vi "XPS_single_axis_control.vi"() -> ()   [LabVIEW 2015]
panel:
  in  "STOP?":bool=TRUE
  out "Current Position":dbl format="%#_13g"
  out "Axis One Position":dbl(graph)
  in  "Target Position":dbl format="%#_13g"
  in  "Group Name":string
  in  "IP Address":string
  # "IP Address of the XPS controller\nis fixed to 192.168.1.43"
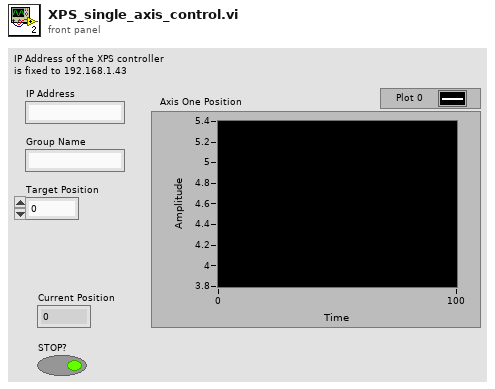
[diagram p1: front panel]
types:
  T1 = cluster{"connection TCP":refnum<k5>, "LogTo File":bool, "Log File refnum":refnum<file>, "no error if error log":bool}
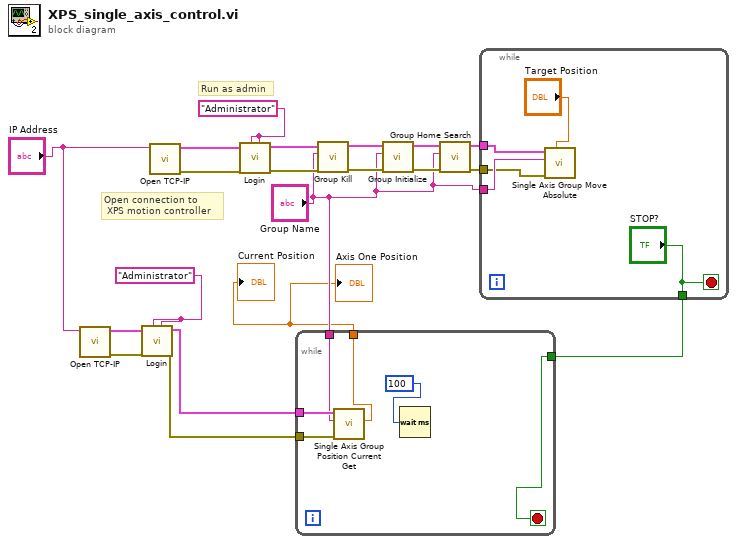
[diagram p0: block diagram]
diagram:
  w6 = "Administrator"
  w19 = "Administrator"
  # "Run as admin"
  # "Open connection to\n XPS motion controller"
  n1 = call <userlib>:"Open TCP-IP.vi"("IP address"="IP Address") -> ("error out"=w7:errorcluster, "Connection ID"=w8:T1)  [unwired: 8 in, 1 out]
  n2 = call <userlib>:"Login.vi"("Password"=w6, "User"=w6, "error in (no error)"=w7, "connection ID in"=w8) -> ("error out"=w4:errorcluster, "connection ID out"=w5:T1)  [unwired: 5 in, 1 out]
  n3 = call <userlib>:"Open TCP-IP.vi"("IP address"="IP Address") -> ("error out"=w14:errorcluster, "Connection ID"=w20:T1)  [unwired: 8 in, 1 out]
  n4 = call <userlib>:"Login.vi"("Password"=w19, "User"=w19, "error in (no error)"=w14, "connection ID in"=w20) -> ("error out"=w13:errorcluster, "connection ID out"=w18:T1)  [unwired: 5 in, 1 out]
  n5 = call <userlib>:"Group Kill.vi"("error in (no error)"=w13, "Group Name (250 c max)"="Group Name", "connection ID in"=w18) -> ("error out"=w12:errorcluster, "connection ID out"=w17:T1)  [unwired: 6 in, 1 out]
  n6 = call <userlib>:"Group Initialize.vi"("error in (no error)"=w12, "Group Name (250 c max)"="Group Name", "connection ID in"=w17) -> ("error out"=w11:errorcluster, "connection ID out"=w16:T1)  [unwired: 6 in, 1 out]
  n7 = call <userlib>:"Group Home Search.vi"("error in (no error)"=w11, "Group Name (250 c max)"="Group Name", "connection ID in"=w16) -> ("error out"=w10:errorcluster, "connection ID out"=w15:T1)  [unwired: 6 in, 1 out]
  n8 = while {
    tunnel: w15 -> [w25]
    tunnel: w10 -> [w23]
    tunnel: "Group Name" -> [w24]
    tunnel: ["STOP?"] -> w1
    stop <- "STOP?" stop-if-true
    n9 = call <userlib>:"Single Axis Group Move Absolute.vi"("Target Position (units)"="Target Position", "error in (no error)"=w23, "SingleAxis Group  Name (250 c max)"=w24, "connection ID in"=w25) -> ()  [unwired: 5 in, 3 out]
  }
  n10 = while {
    tunnel: w5 -> [w31]
    tunnel: w4 -> [w30]
    tunnel: "Group Name" -> [w29]
    tunnel: [w27] -> w2
    tunnel: w1 -> [w26]
    stop <- w26 stop-if-true
    n11 = call <userlib>:"Single Axis Group Position Current Get.vi"("error in (no error)"=w30, "SingleAxis Group  Name (250 c max)"=w29, "connection ID in"=w31) -> ("Current Position (units)"=w27:dbl)  [unwired: 5 in, 3 out]
    n12 = Wait (ms)(milliseconds to wait=100) -> ()  [unwired: 1 out]
  }
  "Axis One Position" <- w2
  "Current Position" <- w2
